vi "DQMH_close modules.vi"(11 "Modules":T1) -> ()   [LabVIEW 2025]
uses:
  Libraries/Data Log/Data Log.lvlib
  Libraries/USB IO/USB IO.lvlib
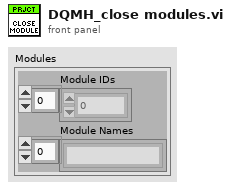
[diagram p1: front panel]
types:
  T1 = cluster{"Module IDs":i32[], "Module Names":string[]}
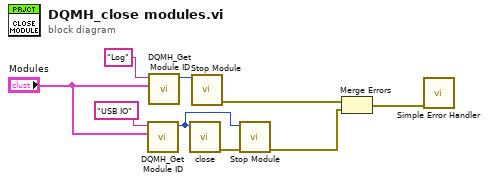
[diagram p0: block diagram]
diagram:
  n1 = call "DQMH_Get Module ID.vi"("Modules"="Modules", "Module Name"="USB IO") -> ("Module ID out"=w5:i32)  [unwired: 9 in]
  n2 = call "DQMH_Get Module ID.vi"("Modules"="Modules", "Module Name"="Log") -> ("Module ID out"=w9:i32)  [unwired: 9 in]
  n3 = call "close.vi"("Module ID"=w5) -> ("error out"=w4:errorcluster)  [unwired: 10 in]
  n4 = call "Stop Module.vi"("Module ID"=w9) -> ("error out"=w3:errorcluster)  [unwired: 10 in]
  n5 = call "Stop Module.vi"("error in"=w4, "Module ID"=w5) -> ("error out"=w2:errorcluster)  [unwired: 9 in]
  n6 = Merge Errors(w3, w2) -> (w1:errorcluster)
  n7 = call <vilib>:"Simple Error Handler.vi"("error in (no error)"=w1) -> ()  [unwired: 4 in, 5 out]
